vi "PopulateQualifiedNamesToPathsList.vi"(8 "error in (no error)":errorcluster, 11 "CDependencyList in":refnum<class "CDependencyList.lvclass">) -> (0 "error out":errorcluster, 3 "CDependencyList out":refnum<class "CDependencyList.lvclass">)   [LabVIEW 2020, in "DependencyInspection.lvlib" / "CDependencyList.lvclass"]
uses:
  CDependencyList.lvclass
  QualifiedNamesToPathsMap.ctl
  CDependencyList.lvclass/CDependencyList.ctl
  obj/Addons/LabVIEWObjectInterfaces.lvlibp/LabVIEWObjectInterfaces/ILabVIEWItem/ILabVIEWItem.lvclass
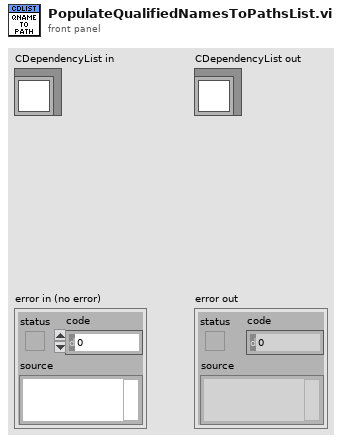
[diagram p1: front panel]
types:
  T1 = typedef "DependencyInspection.lvlib/CDependencyList.lvclass/QualifiedNamesToPathsMap.ctl" = map{string, string}
  T2 = typedef "DependencyInspection.lvlib/CDependencyList.lvclass/DependencyList.ctl" = map{string, refnum<class "ILabVIEWItem.lvclass">}
  T3 = typedef "DependencyInspection.lvlib/CDependencyList.lvclass/QualifiedNamesToPathsMapRef.ctl" = refnum<data-value>
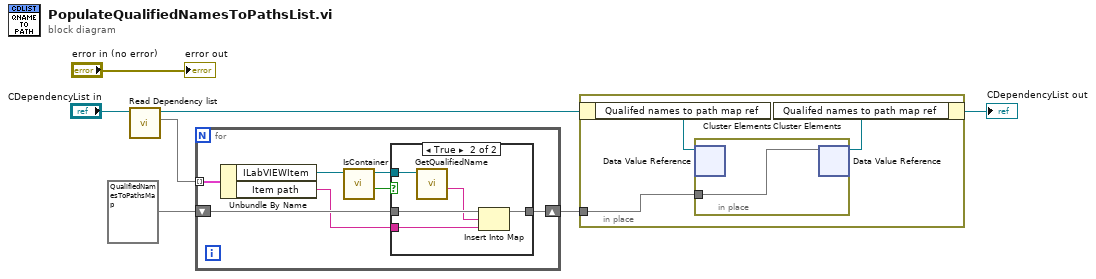
[diagram p0: block diagram]
diagram:
  n1 = call-dynamic "Read Dependency list.vi"("CDependencyList in"="CDependencyList in") -> ("Dependency List"=w5:T2, "CDependencyList out"=w3:refnum<class "CDependencyList.lvclass">)  [unwired: 9 in]
  n2 = for {
    tunnel: w5 -> [w14] mode=indexing
    shift-right: [w8] -> w2
    shift-left: T1 {} -> [w11]
    n3 = Unbundle By Name(w14) -> ("ILabVIEWItem"=w13:refnum<class "ILabVIEWItem.lvclass">, "Item path"=w10:string)
    n4 = call-dynamic "IsContainer.vi"("ILabVIEWItem in"=w13) -> ("Is container?"=w9:bool, "ILabVIEWItem out"=w12:refnum<class "ILabVIEWItem.lvclass">)  [unwired: 8 in, 1 out]
    n5 = case shown="True" w9 {
      tunnel: w12 -> [_ w17]
      tunnel: w11 -> [w15 w20]
      tunnel: w10 -> [_ w19]
      tunnel: [w15 w18] -> w8
      frame False {
      }
      frame True {
        n6 = call-dynamic "GetQualifiedName.vi"("ILabVIEWItem in"=w17) -> ("Qualified name"=w16:string)  [unwired: 8 in, 2 out]
        n7 = Insert Into Map(map in=w20, key=w16, value=w19) -> (map out=w18:T1)  [unwired: 2 out]
      }
    }
  }
  n8 = in-place {
    in-place-border: w2 -> [w21]
    n9 = in-place-cluster #1(w3) -> ("Qualifed names to path map ref"=w23:T3)
    n10 = in-place {
      in-place-border: w21 -> [w24]
      n11 = in-place-dvr #2(w23) -> ()  [unwired: 2 out]
      n12 = in-place-dvr #2(w24) -> (w22:T3)  [unwired: 1 out]
    }
    n13 = in-place-cluster #1("Qualifed names to path map ref"=w22) -> (→"CDependencyList out":refnum<class "CDependencyList.lvclass">)
  }
  "error out" <- "error in (no error)"
